vi "Write gen for DF.vi"(8 "error in (no error)":errorcluster, 10 "gen for DF":bool, 11 "device_type in":refnum<class "device_type.lvclass">) -> (0 "error out":errorcluster, 3 "device_type out":refnum<class "device_type.lvclass">)   [LabVIEW 2021, in "device_type.lvclass"]
uses:
  device_type.lvclass
  device_type.lvclass/device_type.ctl
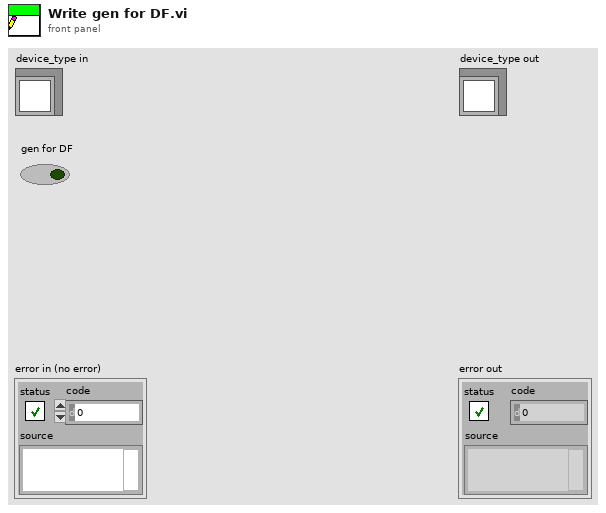
[diagram p1: front panel]
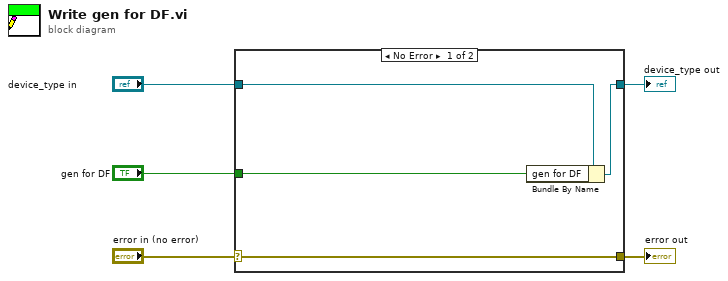
[diagram p0: block diagram]
diagram:
  n1 = case shown="No Error" "error in (no error)" {
    selector: "error in (no error)" -> [w9 w10]
    tunnel: [w9 w10] -> w4
    tunnel: [w7 w11] -> w2
    tunnel: "device_type in" -> [w8 w11]
    tunnel: "gen for DF" -> [w6 _]
    frame No Error {
      n2 = Bundle By Name(cluster=w8, "gen for DF"=w6) -> (w7:refnum<class "device_type.lvclass">)
    }
    frame Error {
    }
  }
  "error out" <- w4
  "device_type out" <- w2
